vi "testing.vi"() -> ()   [LabVIEW 2011]
panel:
  out "Error Array":string[](array[string])
  out "Query Array":string[](array[string])
  out "VISA Out":refnum<visa-resource-name>
  in  "VISA In":refnum<visa-resource-name>
  out "error out":errorcluster
  in  "error in (no error)":errorcluster
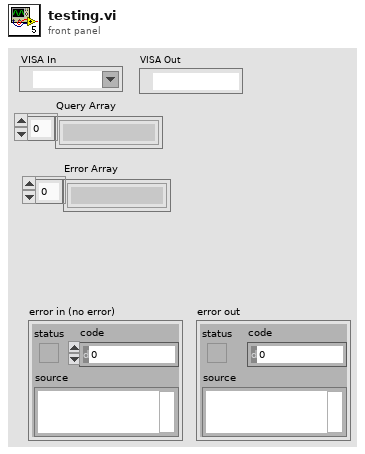
[diagram p1: front panel]
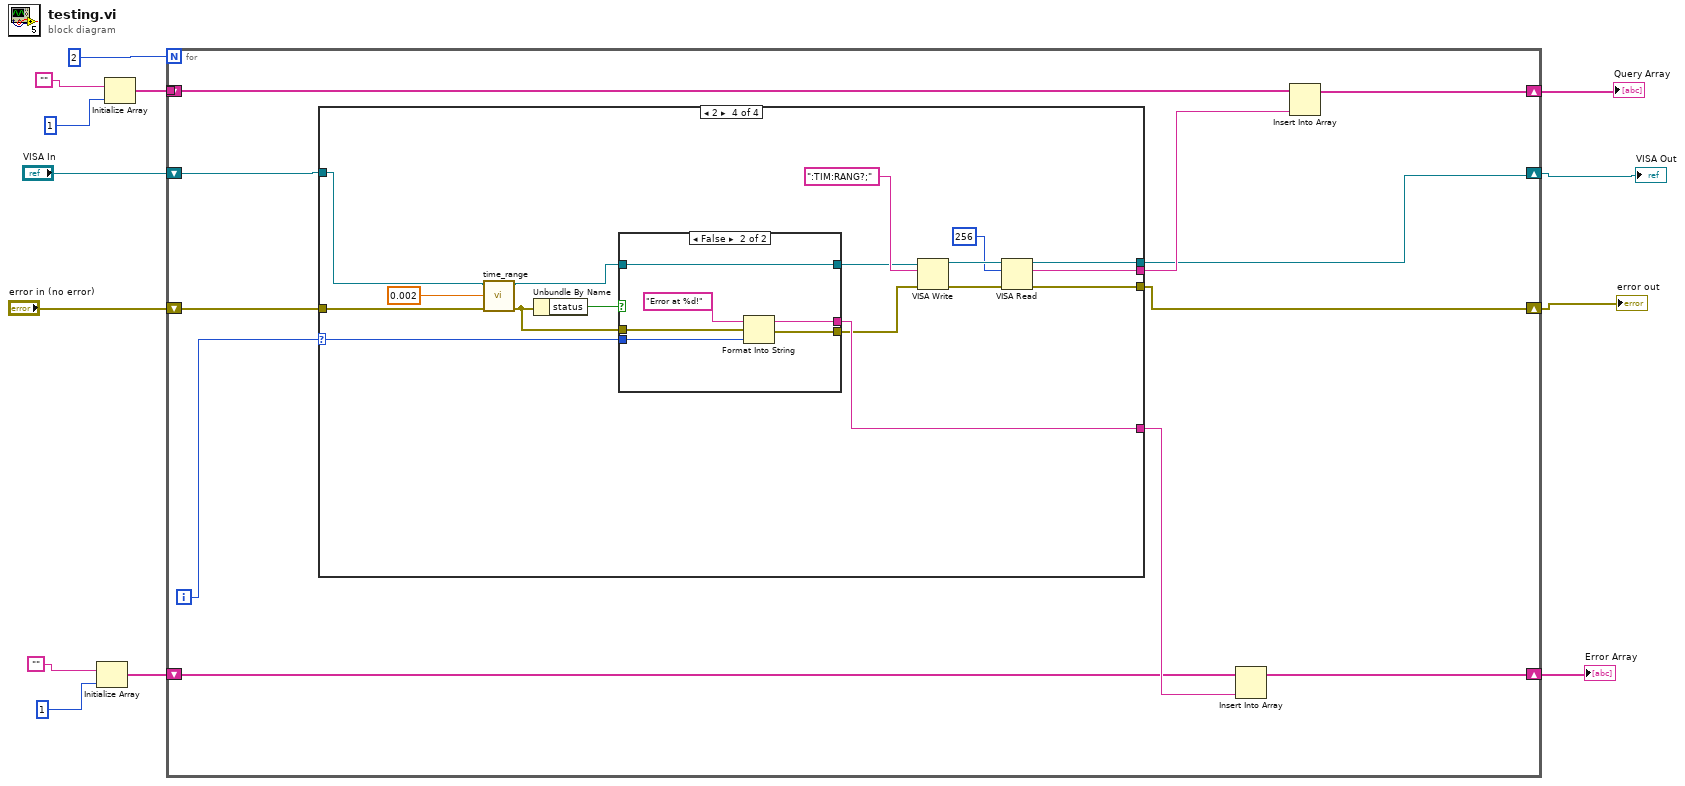
[diagram p0: block diagram]
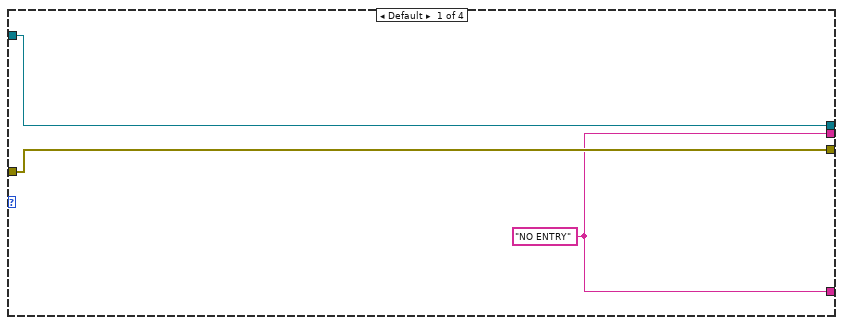
[diagram p2: hidden frame]
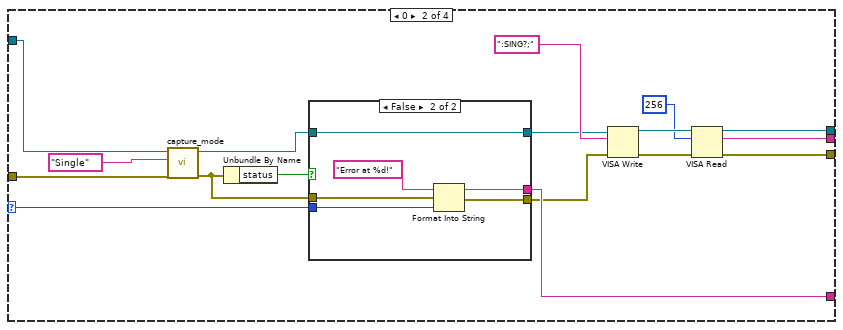
[diagram p3: hidden frame]
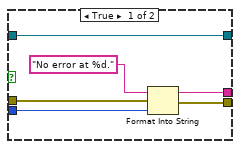
[diagram p4: hidden frame]
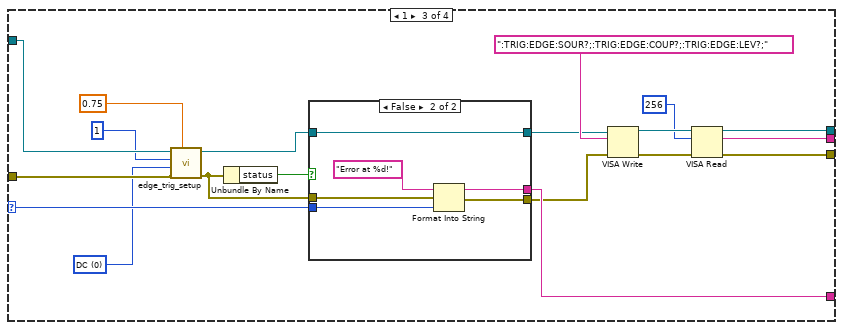
[diagram p5: hidden frame]
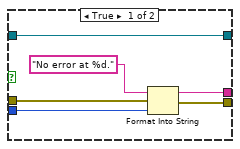
[diagram p6: hidden frame]
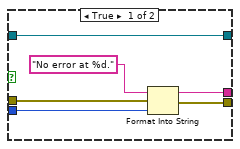
[diagram p7: hidden frame]
diagram:
  n1 = Initialize Array("", 1) -> (w8:string[])
  n2 = Initialize Array("", 1) -> (w5:string[])
  n3 = for {
    N: 2 -> [_]
    shift-right: [w19] -> w2
    shift-left: w8 -> [w20]
    tunnel: w5 -> [w18]
    shift-right: [w16] -> w1
    shift-left: _ -> [_]
    shift-right: [w15] -> w3
    shift-left: "error in (no error)" -> [w22]
    shift-right: [w14] -> w4
    shift-left: "VISA In" -> [w23]
    i -> [w24]
    n4 = case shown="2" w24 {
      selector: w24 -> [_ w40 w74 w103]
      tunnel: w23 -> [w27 w44 w61 w90]
      tunnel: w22 -> [w26 w43 w62 w91]
      tunnel: [w25 w39 w73 w102] -> w21
      tunnel: [w25 w30 w66 w95] -> w17
      tunnel: [w27 w29 w65 w94] -> w14
      tunnel: [w26 w28 w64 w93] -> w15
      frame Default {
        w25 = "NO ENTRY"
      }
      frame 0 {
        n5 = call "capture_mode.vi"("error in (no error)"=w43, "Capture Mode"="Single", "VISA In"=w44) -> ("error out"=w37:errorcluster, "VISA Out"=w38:refnum<visa-resource-name>)  [unwired: 7 in]
        n6 = Unbundle By Name(w37) -> ("status"=w41:bool)
        n7 = case shown="False" w41 {
          tunnel: w40 -> [w49 w55]
          tunnel: [w48 w54] -> w39
          tunnel: w38 -> [w47 w53]
          tunnel: [w47 w53] -> w35
          tunnel: w37 -> [w46 w52]
          tunnel: [w45 w51] -> w34
          frame True {
            n8 = Format Into String(initial string="No error at %d.", error in=w46, w49) -> (resulting string=w48:string, error out=w45:errorcluster)  [unwired: 1 in]
          }
          frame False {
            n9 = Format Into String(initial string="Error at %d!", error in=w52, w55) -> (resulting string=w54:string, error out=w51:errorcluster)  [unwired: 1 in]
          }
        }
        n10 = VISA Write(VISA resource name=w35, write buffer=":SING?;", error in (no error)=w34) -> (VISA resource name out=w33:refnum<visa-resource-name>, error out=w32:errorcluster)  [unwired: 1 out]
        n11 = VISA Read(VISA resource name=w33, byte count=u32 256, error in (no error)=w32) -> (VISA resource name out=w29:refnum<visa-resource-name>, read buffer=w30:string, error out=w28:errorcluster)  [unwired: 1 out]
      }
      frame 1 {
        w58 = u32 0 items=["DC", "AC"] ("Coupling")
        n12 = call "edge_trig_setup.vi"("Tigger Level"=0.75, "error in (no error)"=w62, "Coupling"=w58, "Channel"=u32 1, "VISA In"=w61) -> ("error out"=w63:errorcluster, "VISA Out"=w60:refnum<visa-resource-name>)  [unwired: 5 in]
        n13 = Unbundle By Name(w63) -> ("status"=w75:bool)
        n14 = case shown="False" w75 {
          tunnel: w74 -> [w80 w86]
          tunnel: [w79 w85] -> w73
          tunnel: w60 -> [w78 w84]
          tunnel: [w78 w84] -> w71
          tunnel: w63 -> [w77 w83]
          tunnel: [w76 w82] -> w70
          frame True {
            n15 = Format Into String(initial string="No error at %d.", error in=w77, w80) -> (resulting string=w79:string, error out=w76:errorcluster)  [unwired: 1 in]
          }
          frame False {
            n16 = Format Into String(initial string="Error at %d!", error in=w83, w86) -> (resulting string=w85:string, error out=w82:errorcluster)  [unwired: 1 in]
          }
        }
        n17 = VISA Write(VISA resource name=w71, write buffer=":TRIG:EDGE:SOUR?;:TRIG:EDGE:COUP?;:TRIG:EDGE:LEV?;", error in (no error)=w70) -> (VISA resource name out=w69:refnum<visa-resource-name>, error out=w68:errorcluster)  [unwired: 1 out]
        n18 = VISA Read(VISA resource name=w69, byte count=u32 256, error in (no error)=w68) -> (VISA resource name out=w65:refnum<visa-resource-name>, read buffer=w66:string, error out=w64:errorcluster)  [unwired: 1 out]
      }
      frame 2 {
        n19 = call "time_range.vi"("error in (no error)"=w91, "Time Range"=0.002, "VISA In"=w90) -> ("error out"=w92:errorcluster, "VISA Out"=w89:refnum<visa-resource-name>)  [unwired: 7 in]
        n20 = Unbundle By Name(w92) -> ("status"=w104:bool)
        n21 = case shown="False" w104 {
          tunnel: w103 -> [w109 w115]
          tunnel: [w108 w114] -> w102
          tunnel: w89 -> [w107 w113]
          tunnel: [w107 w113] -> w100
          tunnel: w92 -> [w106 w112]
          tunnel: [w105 w111] -> w99
          frame True {
            n22 = Format Into String(initial string="No error at %d.", error in=w106, w109) -> (resulting string=w108:string, error out=w105:errorcluster)  [unwired: 1 in]
          }
          frame False {
            n23 = Format Into String(initial string="Error at %d!", error in=w112, w115) -> (resulting string=w114:string, error out=w111:errorcluster)  [unwired: 1 in]
          }
        }
        n24 = VISA Write(VISA resource name=w100, write buffer=":TIM:RANG?;", error in (no error)=w99) -> (VISA resource name out=w98:refnum<visa-resource-name>, error out=w97:errorcluster)  [unwired: 1 out]
        n25 = VISA Read(VISA resource name=w98, byte count=u32 256, error in (no error)=w97) -> (VISA resource name out=w94:refnum<visa-resource-name>, read buffer=w95:string, error out=w93:errorcluster)  [unwired: 1 out]
      }
    }
    n26 = Insert Into Array(array=w20, new element=w21) -> (w19:string[])  [unwired: 1 in]
    n27 = Insert Into Array(array=w18, new element=w17) -> (w16:string[])  [unwired: 1 in]
  }
  "error out" <- w3
  "VISA Out" <- w4
  "Error Array" <- w2
  "Query Array" <- w1
